vi "Tree_Init.vi"(0 "object in":refnum<class "Tree.lvclass">, 2 "Root":refnum<class "Node.lvclass">, 5 "Error In":errorcluster) -> (14 "object out":refnum<class "Tree.lvclass">, 19 "Error Out":errorcluster)   [LabVIEW 2024, in "Tree.lvclass"]
uses:
  Tree.lvclass
  Tree.lvclass/Tree.ctl
  Node_class/Node.lvclass
panel:
  # "Connector Pane"
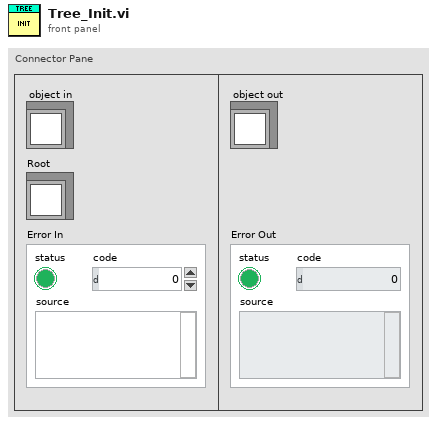
[diagram p1: front panel]
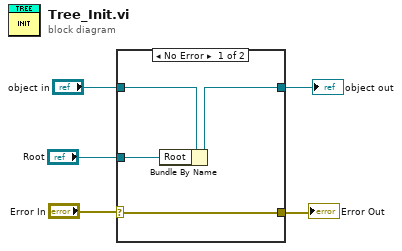
[diagram p0: block diagram]
diagram:
  n1 = case shown="No Error" "Error In" {
    selector: "Error In" -> [w7 w10]
    tunnel: "object in" -> [w9 w11]
    tunnel: [w8 w11] -> w4
    tunnel: [w7 w10] -> w2
    tunnel: "Root" -> [w6 _]
    frame No Error {
      n2 = Bundle By Name(cluster=w9, "Root"=w6) -> (w8:refnum<class "Tree.lvclass">)
    }
    frame Error {
    }
  }
  "object out" <- w4
  "Error Out" <- w2
